vi "Get DataSet Ref.vi"(8 "error in (no error)":errorcluster caption="错误输入（无错误）", 11 "OleDBClass 输入":refnum<class "OleDBClass.lvclass"> caption="DNL_LabVIEW Object in") -> (0 "error out":errorcluster caption="错误输出", 2 "DataSet":refnum<k24>, 3 "OleDBClass 输出":refnum<class "OleDBClass.lvclass"> caption="DNL_LabVIEW Object out")   [LabVIEW 2012, in "OleDBClass.lvclass"]
uses:
  OleDBClass.lvclass
  System.Data
  OleDBClass.lvclass/OleDBClass.ctl
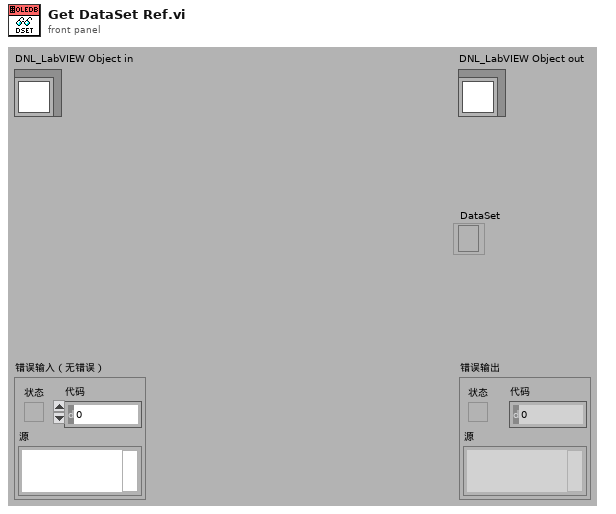
[diagram p1: front panel]
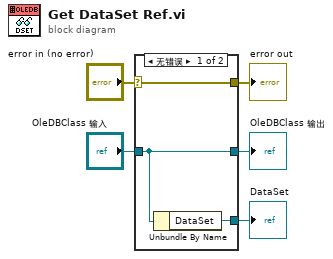
[diagram p0: block diagram]
diagram:
  n1 = case shown="无错误" "error in (no error)" {
    selector: "error in (no error)" -> [w8 w10]
    tunnel: [w8 w10] -> w4
    tunnel: [w7 w9] -> w2
    tunnel: "OleDBClass 输入" -> [w7 w9]
    tunnel: [w6 _] -> w1
    frame No Error {
      n2 = Unbundle By Name(w7) -> ("DataSet"=w6:refnum<k24>)
    }
    frame Error {
    }
  }
  "error out" <- w4
  "OleDBClass 输出" <- w2
  "DataSet" <- w1
